vi "Is subVI.vi"() -> (0 "Is subVI?":bool)   [LabVIEW 2018]
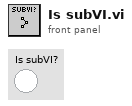
[diagram p1: front panel]
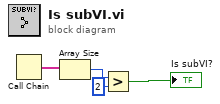
[diagram p0: block diagram]
diagram:
  n1 = Call Chain() -> (call chain=w2:string[])
  n2 = Array Size(array=w2) -> (size(s)=w3:i32)
  n3 = Greater?(x=w3, y=2) -> (0:→"Is subVI?":bool)
